vi "VRM Calculate Sweep Rates.vi"(8 "error in (no error)":errorcluster, 9 "Sweep rate (T/min)":dbl, 10 "Target Field (T)":dbl[](array[numeric]), 11 "Initial Field (T)":dbl[](array[numeric])) -> (0 "error out":errorcluster, 1 "time (min)":dbl, 3 "Sweep Rate Field (T/min)":dbl[](array[numeric]))   [LabVIEW 2019, in "Instrument.OxfordVRM.lvclass"]
uses:
  Instrument.OxfordVRM.lvclass
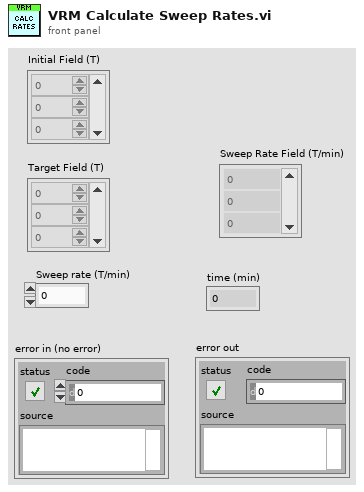
[diagram p1: front panel]
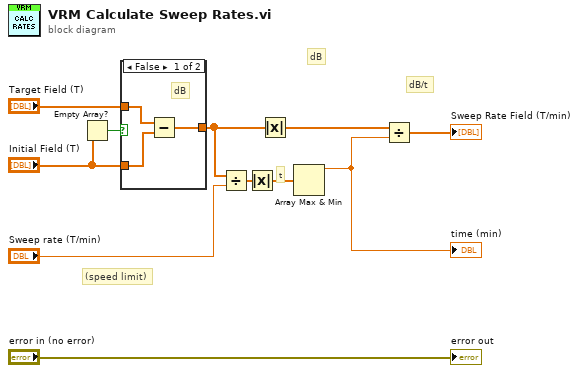
[diagram p0: block diagram]
diagram:
  # "dB/t"
  # "dB"
  # "(speed limit)"
  # "t"
  n1 = Empty Array?(array="Initial Field (T)") -> (empty?=w1:bool)
  n2 = case shown="False" w1 {
    tunnel: [w14 w15] -> w5
    tunnel: "Target Field (T)" -> [w13 w15]
    tunnel: "Initial Field (T)" -> [w12 _]
    frame False {
      # "dB"
      n3 = Subtract(x=w13, y=w12) -> (x-y=w14:dbl[])
    }
    frame True {
    }
  }
  n4 = Divide(x=w5, y="Sweep rate (T/min)") -> (x/y=w10:dbl[])
  n5 = Absolute Value(x=w10) -> (abs(x)=w7:dbl[])
  n6 = Absolute Value(x=w5) -> (abs(x)=w6:dbl[])
  n7 = Array Max & Min(array=w7) -> (max value=w9:dbl)  [unwired: 3 out]
  "time (min)" <- w9
  n8 = Divide(x=w6, y=w9) -> (x/y=→"Sweep Rate Field (T/min)":dbl[])
  "error out" <- "error in (no error)"
